vi "throttle.vi"() -> ()   [LabVIEW 2012]
panel:
  out "Throttle":bool
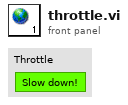
[diagram p1: front panel]
diagram:
